vi "Advantech DAQ Get Data.vi"(8 "Error In":errorcluster, 11 "TC Coefficients":T2) -> (0 "Error Out":errorcluster, 3 "Advantech":T1, 5 "Avantech DAQ":string[][](array[string]), 7 "Parametric DBL Data":dbl[](array[numeric]))   [LabVIEW 2019]
doc: "This VI sets the correct device and associated properties..It then reads the data from the device."
uses:
  Trunk/Utility/Type Definitions/UTILITY TC Coefficients.ctl
  Type Definitions/Advantech DAQ.ctl
  <userlib>/DAQNavi Polymorphic VI/read/DAQNavi Read (Analog 1D DBL NChan 1Samp).vi
panel:
  out "Raw Data":dbl[](array[numeric])
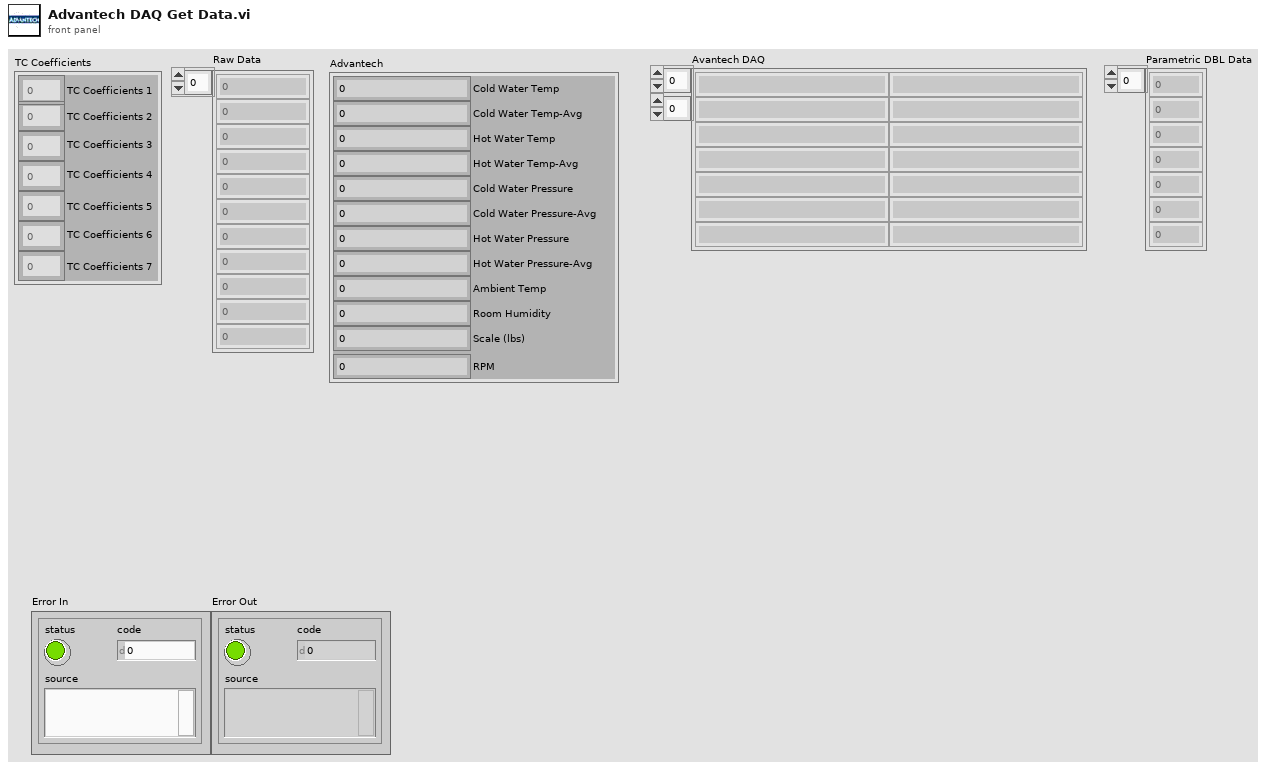
[diagram p1: front panel]
types:
  T1 = typedef "Advantech DAQ.ctl" = cluster{"Cold Water Pressure":dbl, "Hot Water Pressure":dbl, "Cold Water Temp":dbl, "Hot Water Temp":dbl, "Ambient Temp":dbl, "Room Humidity":dbl, "Scale (lbs)":dbl, "RPM":dbl, "Cold Water Temp-Avg":dbl, "Hot Water Temp-Avg":dbl, "Cold Water Pressure-Avg":dbl, "Hot Water Pressure-Avg":dbl}
  T2 = typedef "UTILITY TC Coefficients.ctl" = cluster{"TC Coefficients 1":dbl[], "TC Coefficients 2":dbl[], "TC Coefficients 3":dbl[], "TC Coefficients 4":dbl[], "TC Coefficients 5":dbl[], "TC Coefficients 6":dbl[], "TC Coefficients 7":dbl[]}
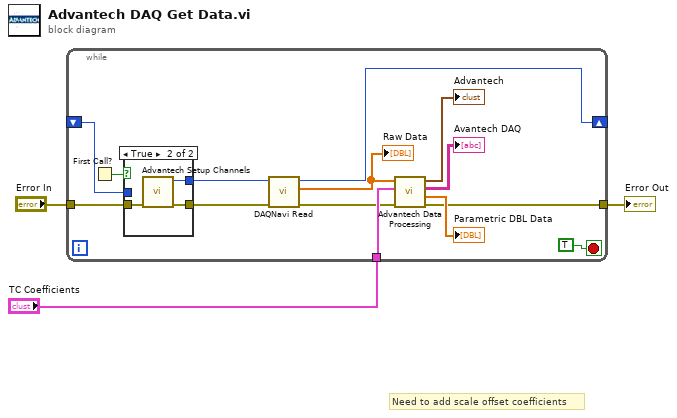
[diagram p0: block diagram]
diagram:
  # "Need to add scale offset coefficients"
  n1 = while {
    tunnel: "TC Coefficients" -> [w17]
    tunnel: [w11] -> w2
    tunnel: "Error In" -> [w10]
    shift-right: [w7] -> _
    shift-left: _ -> [w6]
    stop <- TRUE stop-if-true
    n2 = First Call?() -> (First Call?: T/F=w15:bool)
    n3 = case shown="True" w15 {
      tunnel: [w18 w22] -> w8
      tunnel: w10 -> [w19 w21]
      tunnel: [w19 w20] -> w9
      tunnel: w6 -> [w18 _]
      frame False {
      }
      frame True {
        n4 = call "Advantech Setup Channels.vi"("error in (no error)"=w21) -> ("error out"=w20:errorcluster, "task out"=w22:i32)  [unwired: 9 in]
      }
    }
    n5 = call-poly <userlib>:"DAQNavi Read.vi"("error in (no error)"=w9, "task in"=w8) -> ("error out"=w5:errorcluster, "data"=w4:dbl[], "task out"=w7:i32)  [unwired: 7 in]
    "Raw Data" <- w4
    n6 = call "Advantech Data Processing.vi"("Error In"=w5, "TC Coefficients"=w17, "Raw Data"=w4) -> ("Error Out"=w11:errorcluster, "Advantech Data Output"=→"Parametric DBL Data":dbl[], "Advantech Data List Headers"=→"Avantech DAQ":string[][], "Advantech"=→"Advantech":T1)  [unwired: 5 in]
  }
  "Error Out" <- w2
